vi "ccdDiscover.vi"(8 "error in (no error)":errorcluster, 11 "CCD in":refnum<class "CCD.lvclass">) -> (0 "error out":errorcluster, 2 "CCD count":T1, 3 "CCD out":refnum<class "CCD.lvclass">)   [LabVIEW 2023, in "CCD.lvclass"]
uses:
  CCD.lvclass
  CCD.lvclass/CCD.ctl
  ab6658d7-4a50-4d30-a470-11fb8c9dbb3f.vi
  Communicator/Communicator.lvclass
  d18f7746-8b9c-45eb-8a46-5cc64a405b53.vi
  GenericDevice/GenericDevice.lvclass
  ccdCount.ctl
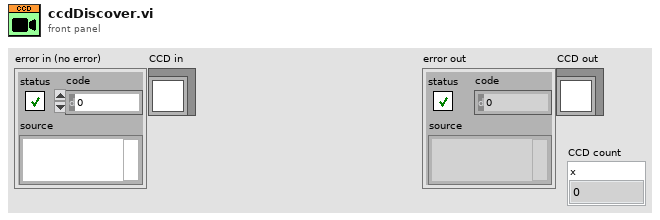
[diagram p1: front panel]
types:
  T1 = typedef "CCD.lvclass/ccdCount.ctl" = cluster{"x":i32}
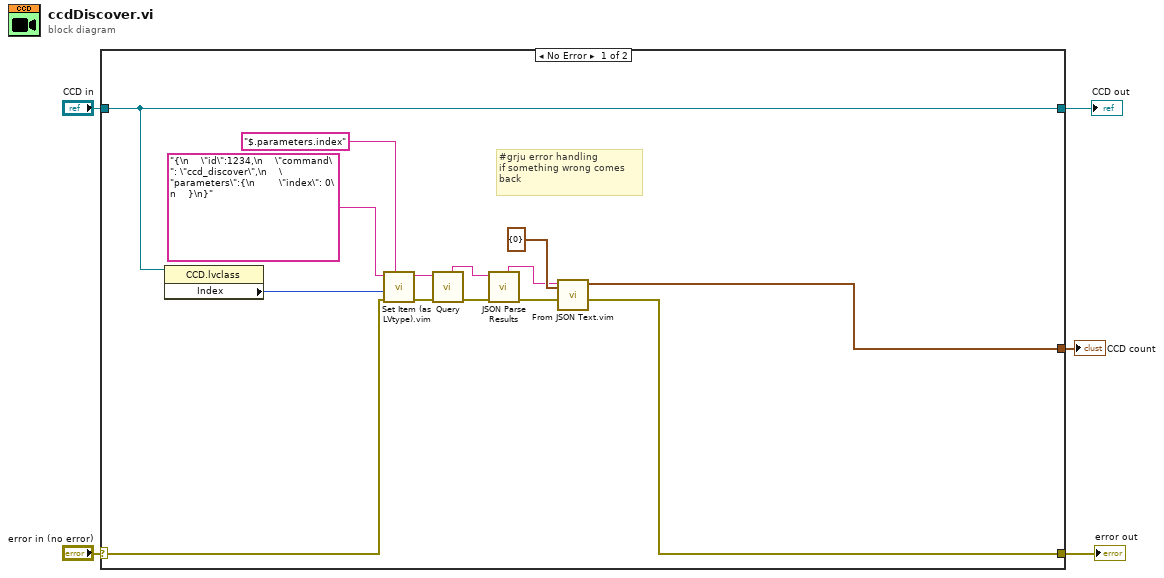
[diagram p0: block diagram]
diagram:
  n1 = case shown="No Error" "error in (no error)" {
    selector: "error in (no error)" -> [w15 w21]
    tunnel: [w12 w21] -> w4
    tunnel: [w17 w20] -> w2
    tunnel: "CCD in" -> [w17 w20]
    tunnel: [w14 _] -> w1
    frame No Error {
      # "#grju error handling\nif something wrong comes\nback"
      n2 = property class="CCD.lvclass"(reference=w17) -> ("Index"=w16:i32)  [unwired: 1 in, 2 out]
      n3 = call "Set Item (as LVtype).vim"("$Path or Item Name"="$.parameters.index", "error in (no error)"=w15, "Anything"=w16, "JSON"="{\n    \"id\":1234,\n    \"command\": \"ccd_discover\",\n    \"parameters\":{\n        \"index\": 0\n    }\n}") -> ("error out"=w9:errorcluster, "<JSON>"=w11:string)  [unwired: 4 in, 1 out]
      n4 = call "Query.vi"("error in (no error)"=w9, "String to be sent"=w11) -> ("error out"=w8:errorcluster, "answer from device"=w10:string)  [unwired: 5 in, 3 out]
      n5 = call "JSON Parse Results.vi"("error in (no error)"=w8, "JSON"=w10) -> ("error out"=w13:errorcluster, "results-JSON string"=w6:string)  [unwired: 5 in, 3 out]
      n6 = call "From JSON Text.vim"("Data Type and Default Value"=T1 {"x"=0} ("Numeric"), "error in (no error)"=w13, "JSON"=w6) -> ("error out"=w12:errorcluster, "Data out"=w14:T1)  [unwired: 7 in]
    }
    frame Error {
    }
  }
  "error out" <- w4
  "CCD out" <- w2
  "CCD count" <- w1
